vi "set parameter - array of bytes.vi"(8 "error in (no error)":errorcluster, 9 "value":u8[](array[numeric]), 10 "parameter":u8 format="%x", 11 "channel":u16 format="%x") -> (0 "error out":errorcluster)   [LabVIEW 2024, in "atsj peakcan basic.lvlib"]
doc: "Sets a parameter for a PeakCAN <b>channel</b>."
uses:
  atsj peakcan basic.lvlib
  support/x64/PCANBasic.dll
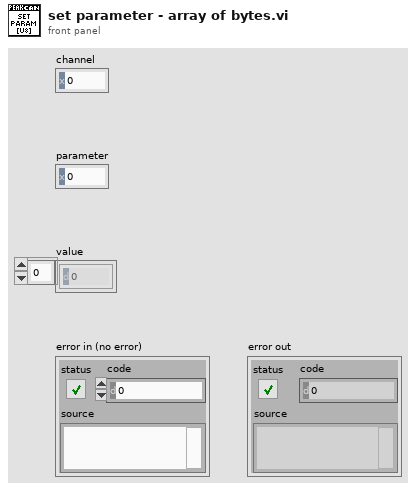
[diagram p1: front panel]
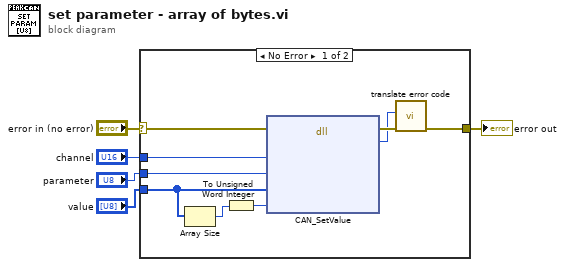
[diagram p0: block diagram]
diagram:
  n1 = case shown="No Error" "error in (no error)" {
    selector: "error in (no error)" -> [w13 w15]
    tunnel: [w14 w15] -> w4
    tunnel: "channel" -> [w10 _]
    tunnel: "parameter" -> [w9 _]
    tunnel: "value" -> [w8 _]
    frame No Error {
      n2 = Array Size(array=w8) -> (size(s)=w7:i32)
      n3 = To Unsigned Word Integer(number=w7) -> (unsigned 16bit integer=w6:u16)
      n4 = dll-call lib="C:/atsj/plateau/atsj-peakcan-basic-for-labview/src/support/x64/PCANBasic.dll" fn="CAN_SetValue" ("set parameter - array of bytes")(error in=w13, "Channel"=w10, "Parameter"=w9, "Buffer"=w8, "BufferLength"=w6) -> (error out=w12:errorcluster, "Status"=w11:u32)  [unwired: 6 in, 1 out]
      n5 = call "translate error code.vi"("error in (no error)"=w12, "error code"=w11) -> ("error out"=w14:errorcluster)  [unwired: 9 in]
    }
    frame Error {
    }
  }
  "error out" <- w4
